vi "PZT Set Position-精调.vi"(8 "Set Position （°/mm）":dbl, 9 "Origin":dbl=5.0, 10 "Range":dbl=10.92, 11 "VISA resource name":refnum<visa-resource-name> caption="VISA资源名称") -> (1 "Set Position-Real （°/mm）":dbl, 2 "Current Position （mm  /  °）":dbl, 3 "VISA资源名称输出":refnum<visa-resource-name>)   [LabVIEW 2014]
panel:
  out "初始运动方向":bool
  out "x > 0?":bool
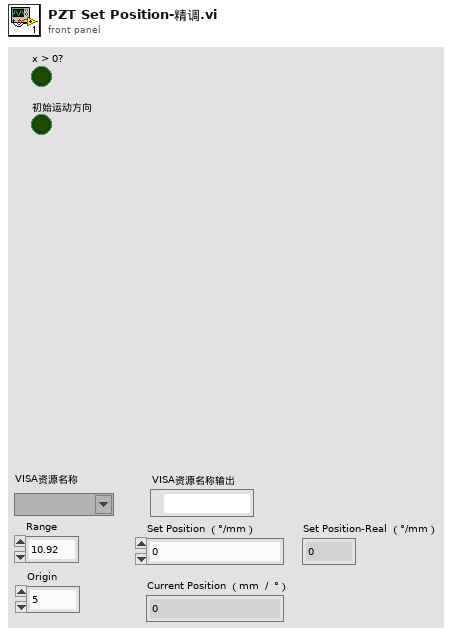
[diagram p1: front panel]
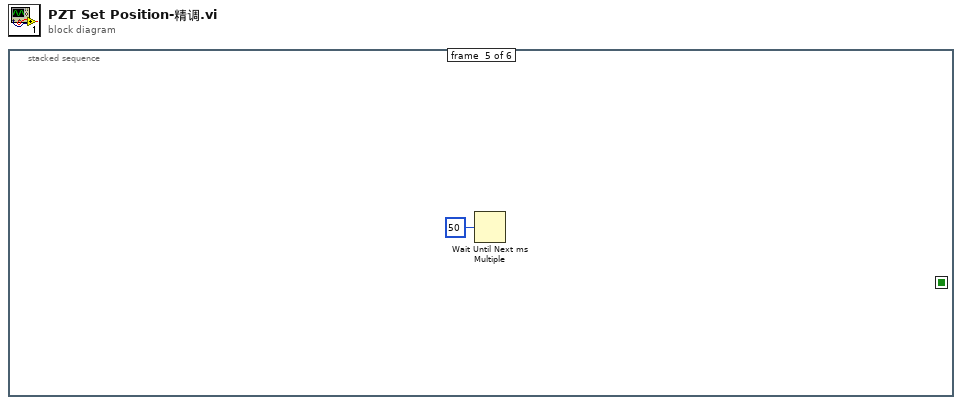
[diagram p0: block diagram]
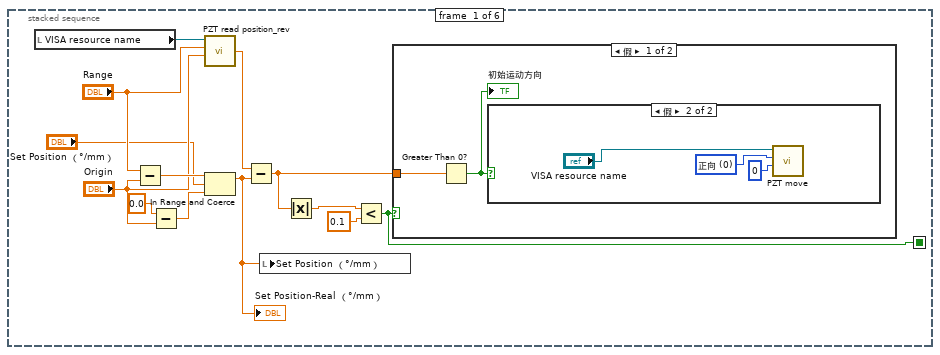
[diagram p2: hidden frame]
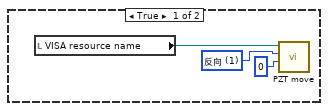
[diagram p3: hidden frame]
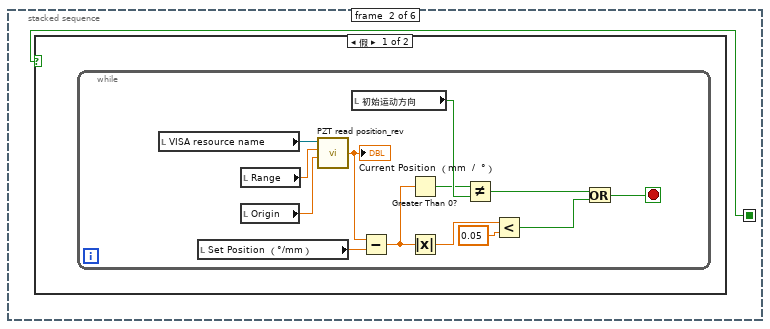
[diagram p5: hidden frame]
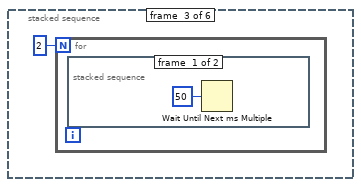
[diagram p7: hidden frame]
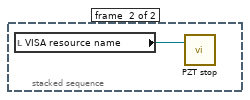
[diagram p8: hidden frame]
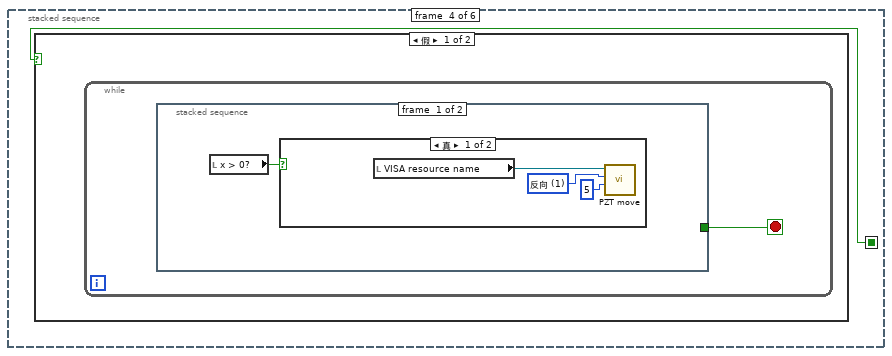
[diagram p9: hidden frame]
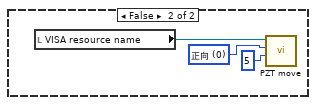
[diagram p10: hidden frame]
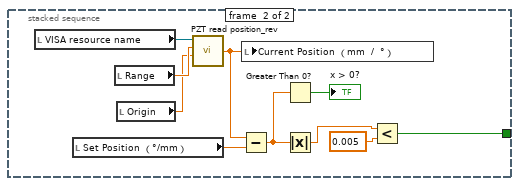
[diagram p11: hidden frame]
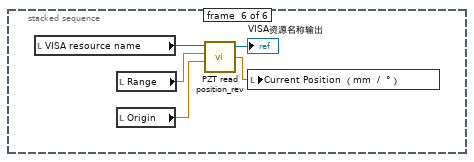
[diagram p13: hidden frame]
diagram:
  n1 = stacked-sequence {
    seq-local: [w9 _ _ _ _ _] -> [_ w22 _ w39 _ _]
    frame #0 {
      n2 = local read "VISA resource name"() -> (w13:refnum<visa-resource-name>)
      n3 = Subtract(x="Range", y="Origin") -> (x-y=w5:dbl)
      n4 = Subtract(x=0.0, y="Origin") -> (x-y=w4:dbl)
      n5 = call "PZT read position_rev.vi"("Origin"="Origin", "Range"="Range", "VISA resource name"=w13) -> ("Current Position （mm  /  °）"=w12:dbl)  [unwired: 1 in, 2 out]
      n6 = In Range and Coerce(upper limit=w5, x="Set Position （°/mm）", lower limit=w4) -> (coerced(x)=w1:dbl)  [unwired: 1 out]
      "Set Position-Real （°/mm）" <- w1
      n7 = Subtract(x=w12, y=w1) -> (x-y=w10:dbl)
      n8 = local write "Set Position （°/mm）"(w1) -> ()
      n9 = Absolute Value(x=w10) -> (abs(x)=w8:dbl)
      n10 = Less?(x=w8, y=0.1) -> (x < y?=w9:bool)
      n11 = case shown="假" w9 {
        tunnel: w10 -> [w14 _]
        frame False {
          n12 = Greater Than 0?(x=w14) -> (x > 0?=w15:bool)
          "初始运动方向" <- w15
          n13 = case shown="假" w15 {
            frame True {
              w18 = u16 1 items=["正向", "反向"] ("移动方向")
              n14 = local read "VISA resource name"() -> (w16:refnum<visa-resource-name>)
              n15 = call "PZT move.vi"("移动步数"=0, "移动方向"=w18, "VISA resource name"=w16) -> ()  [unwired: 1 in, 2 out]
            }
            frame False {
              w20 = u16 0 items=["正向", "反向"] ("移动方向")
              n16 = call "PZT move.vi"("移动步数"=0, "移动方向"=w20, "VISA resource name"="VISA resource name") -> ()  [unwired: 1 in, 2 out]
            }
          }
        }
        frame True {
        }
      }
    }
    frame #1 {
      n17 = case shown="假" w22 {
        frame False {
          n18 = while {
            stop <- w23 stop-if-true
            n19 = local read "VISA resource name"() -> (w35:refnum<visa-resource-name>)
            n20 = local read "Set Position （°/mm）"() -> (w31:dbl)
            n21 = local read "Range"() -> (w34:dbl)
            n22 = local read "Origin"() -> (w33:dbl)
            n23 = call "PZT read position_rev.vi"("Origin"=w33, "Range"=w34, "VISA resource name"=w35) -> ("Current Position （mm  /  °）"=w32:dbl)  [unwired: 1 in, 2 out]
            "Current Position （mm  /  °）" <- w32
            n24 = local read "初始运动方向"() -> (w27:bool)
            n25 = Subtract(x=w32, y=w31) -> (x-y=w28:dbl)
            n26 = Greater Than 0?(x=w28) -> (x > 0?=w26:bool)
            n27 = Absolute Value(x=w28) -> (abs(x)=w30:dbl)
            n28 = Not Equal?(x=w26, y=w27) -> (x != y?=w25:bool)
            n29 = Less?(x=w30, y=0.05) -> (x < y?=w24:bool)
            n30 = Or(x=w25, y=w24) -> (x .or. y?=w23:bool)
          }
        }
        frame True {
        }
      }
    }
    frame #2 {
      n31 = for {
        N: 2 -> [_]
        n32 = stacked-sequence {
          frame #0 {
            n33 = Wait Until Next ms Multiple(millisecond multiple=u32 50 ("毫秒倍数")) -> ()  [unwired: 1 out]
          }
          frame #1 {
            n34 = local read "VISA resource name"() -> (w38:refnum<visa-resource-name>)
            n35 = call "PZT stop.vi"("VISA resource name"=w38) -> ()  [unwired: 1 in, 2 out]
          }
        }
      }
    }
    frame #3 {
      n36 = case shown="假" w39 {
        frame False {
          n37 = while {
            stop <- w40 stop-if-true
            n38 = stacked-sequence {
              tunnel: [_ w50] -> w40
              frame #0 {
                n39 = local read "x > 0?"() -> (w41:bool)
                n40 = case shown="真" w41 {
                  frame True {
                    w44 = u16 1 items=["正向", "反向"] ("移动方向")
                    n41 = local read "VISA resource name"() -> (w42:refnum<visa-resource-name>)
                    n42 = call "PZT move.vi"("移动步数"=5, "移动方向"=w44, "VISA resource name"=w42) -> ()  [unwired: 1 in, 2 out]
                  }
                  frame False {
                    w47 = u16 0 items=["正向", "反向"] ("移动方向")
                    n43 = local read "VISA resource name"() -> (w45:refnum<visa-resource-name>)
                    n44 = call "PZT move.vi"("移动步数"=5, "移动方向"=w47, "VISA resource name"=w45) -> ()  [unwired: 1 in, 2 out]
                  }
                }
              }
              frame #1 {
                n45 = local read "VISA resource name"() -> (w57:refnum<visa-resource-name>)
                n46 = local read "Set Position （°/mm）"() -> (w54:dbl)
                n47 = local read "Range"() -> (w56:dbl)
                n48 = local read "Origin"() -> (w55:dbl)
                n49 = call "PZT read position_rev.vi"("Origin"=w55, "Range"=w56, "VISA resource name"=w57) -> ("Current Position （mm  /  °）"=w48:dbl)  [unwired: 1 in, 2 out]
                n50 = Subtract(x=w48, y=w54) -> (x-y=w53:dbl)
                n51 = local write "Current Position （mm  /  °）"(w48) -> ()
                n52 = Greater Than 0?(x=w53) -> (x > 0?=→"x > 0?":bool)
                n53 = Absolute Value(x=w53) -> (abs(x)=w52:dbl)
                n54 = Less?(x=w52, y=0.005) -> (x < y?=w50:bool)
              }
            }
          }
        }
        frame True {
        }
      }
    }
    frame #4 {
      n55 = Wait Until Next ms Multiple(millisecond multiple=u32 50 ("毫秒倍数")) -> ()  [unwired: 1 out]
    }
    frame #5 {
      n56 = local read "VISA resource name"() -> (w63:refnum<visa-resource-name>)
      n57 = local read "Range"() -> (w62:dbl)
      n58 = local read "Origin"() -> (w61:dbl)
      n59 = call "PZT read position_rev.vi"("Origin"=w61, "Range"=w62, "VISA resource name"=w63) -> ("Current Position （mm  /  °）"=w60:dbl, "VISA资源名称输出"=→"VISA资源名称输出":refnum<visa-resource-name>)  [unwired: 1 in, 1 out]
      n60 = local write "Current Position （mm  /  °）"(w60) -> ()
    }
  }
